vi "Read Temperature.vi"(8 "error in (no error)":errorcluster, 11 "Simple Device in":refnum<class "Simple Device.lvclass">) -> (0 "error out":errorcluster, 2 "Temperature":dbl, 3 "Simple Device out":refnum<class "Simple Device.lvclass">)   [LabVIEW 2020, in "Simple Device.lvclass"]
uses:
  Simple Device.lvclass
  Simple Device.lvclass/Simple Device.ctl
  TALOS/TALOS_PPL.lvlibp
  DeviceSim.lvlibp/DeviceReference/Simple  Virtual Device.lvclass
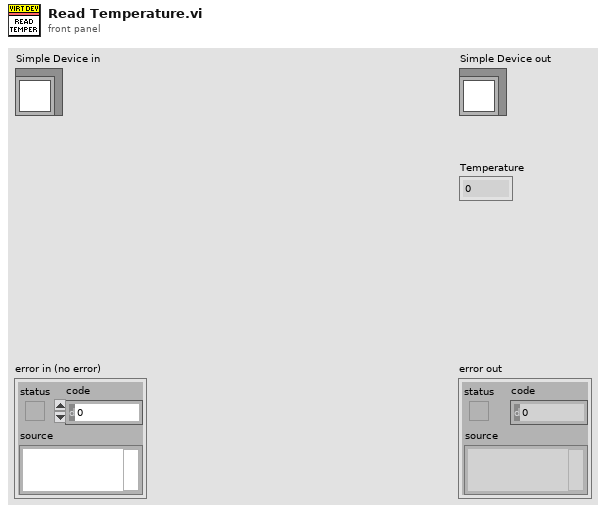
[diagram p1: front panel]
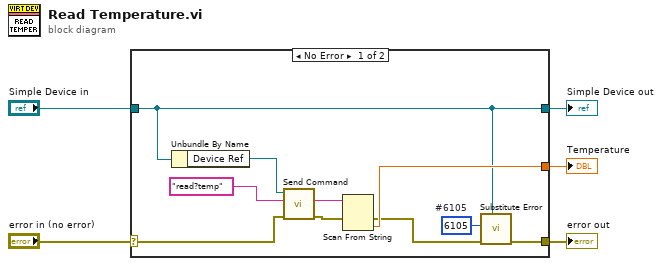
[diagram p0: block diagram]
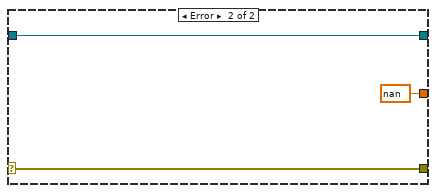
[diagram p2: hidden frame]
diagram:
  n1 = case shown="No Error" "error in (no error)" {
    selector: "error in (no error)" -> [w14 w18]
    tunnel: [w8 w18] -> w4
    tunnel: [w7 w17] -> w2
    tunnel: "Simple Device in" -> [w7 w17]
    tunnel: [w10 nan] -> w1
    frame No Error {
      w6 = 6105  # #6105
      n2 = Unbundle By Name(w7) -> ("Device Ref"=w15:refnum<data-value>)
      n3 = call "Send Command.vi"("error in (no error)"=w14, "Command"="read?temp", "Device Ref in"=w15) -> ("error out"=w11:errorcluster, "Response"=w12:string)  [unwired: 6 in, 1 out]
      n4 = Scan From String(input string=w12, error in=w11) -> (error out=w9:errorcluster, output 1=w10:dbl)  [unwired: 3 in, 2 out]
      n5 = call "Substitute Error.vi"("LabVIEW Object"=w7, "error in (no error)"=w9, "Error Code"=w6) -> ("error out"=w8:errorcluster)  [unwired: 8 in]
    }
    frame Error {
    }
  }
  "error out" <- w4
  "Simple Device out" <- w2
  "Temperature" <- w1
